vi "Static Error Handling.Source Buffer.Write.String.vi"(9 "offset":i32, 10 "string":string, 11 "error in":errorcluster) -> (1 "new offset":i32, 3 "error out":errorcluster)   [LabVIEW 2016, in "Memory Manager.lvlib" / "Static Error Handling.lvlib"]
doc: "Writes <b>string</b> to the <b>error in</b> source buffer at the specified <b>offset</b>."
uses:
  Static Error Handling.lvlib
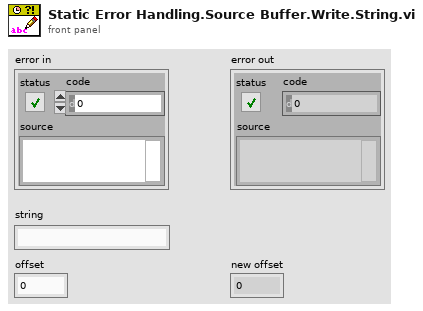
[diagram p1: front panel]
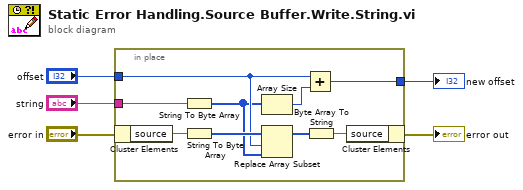
[diagram p0: block diagram]
diagram:
  n1 = in-place {
    in-place-border: "string" -> [w11]
    in-place-border: "offset" -> [w9]
    in-place-border: [w6] -> w2
    n2 = in-place-cluster #1("error in") -> ("source"=w13:string)
    n3 = String To Byte Array(string=w11) -> (unsigned byte array=w8:u8[])
    n4 = String To Byte Array(string=w13) -> (unsigned byte array=w12:u8[])
    n5 = Array Size(array=w8) -> (size(s)=w7:i32)
    n6 = Replace Array Subset(array=w12, new element=w8, index=w9) -> (w10:u8[])
    n7 = Add(x=w9, y=w7) -> (x+y=w6:i32)
    n8 = Byte Array To String(unsigned byte array=w10) -> (string=w14:string)
    n9 = in-place-cluster #1("source"=w14) -> (→"error out":errorcluster)
  }
  "new offset" <- w2
